vi "Log Range.vi"(1 "Max":dbl=2559.999999999547, 2 "Min":dbl=0.2222222222222222, 3 "Number Elements":u32=200) -> (0 "Log Range":dbl[](array[numeric]))   [LabVIEW 2022 SP3]
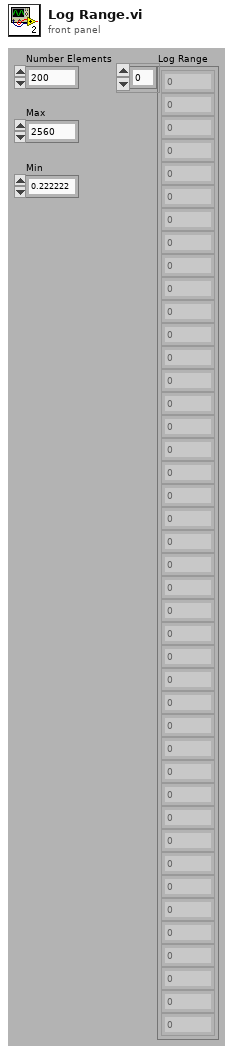
[diagram p1: front panel]
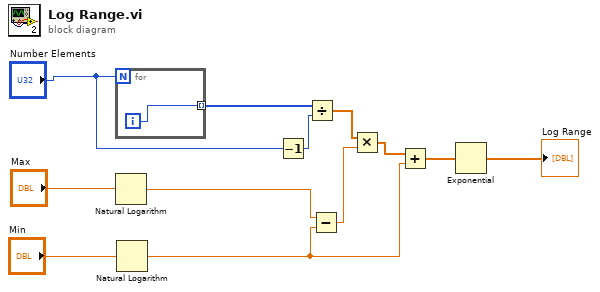
[diagram p0: block diagram]
diagram:
  n1 = for {
    N: "Number Elements" -> [_]
    tunnel: [w13] -> w8 mode=indexing
    i -> [w13]
  }
  n2 = Natural Logarithm(1:"Max") -> (0:w7:dbl)
  n3 = Natural Logarithm(1:"Min") -> (0:w3:dbl)
  n4 = Decrement(x="Number Elements") -> (x-1=w9:u32)
  n5 = Divide(x=w8, y=w9) -> (x/y=w5:dbl[])
  n6 = Subtract(x=w7, y=w3) -> (x-y=w6:dbl)
  n7 = Multiply(x=w5, y=w6) -> (x*y=w4:dbl[])
  n8 = Add(x=w4, y=w3) -> (x+y=w2:dbl[])
  n9 = Exponential(1:w2) -> (0:→"Log Range":dbl[])
